vi "dark int time.vi"(8 "error in (no error)":errorcluster) -> (0 "error out":errorcluster, 1 "Stop and Save":bool, 2 "int time":dbl)   [LabVIEW 2013]
uses:
  <vilib>/Utility/file.llb/Read From Spreadsheet File (DBL).vi
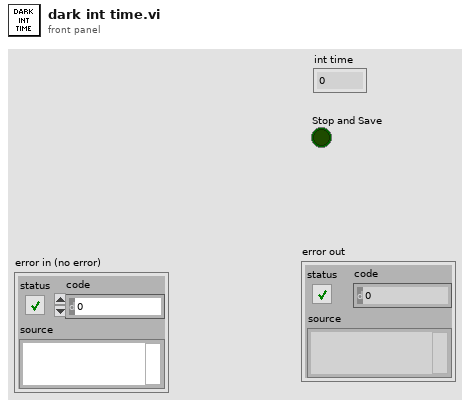
[diagram p1: front panel]
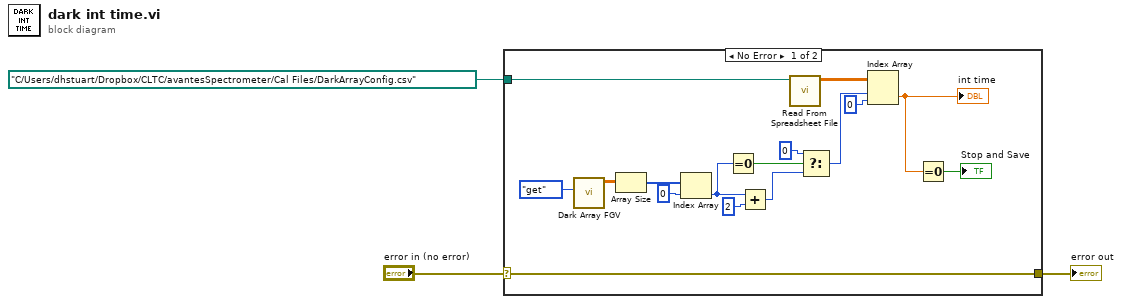
[diagram p0: block diagram]
diagram:
  n1 = case shown="No Error" "error in (no error)" {
    selector: "error in (no error)" -> [w6 w20]
    tunnel: path "C:/Users/dhstuart/Dropbox/CLTC/avantesSpectrometer/Cal Files/DarkArrayConfig.csv" ("file path (dialog if empty)") -> [w19 _]
    tunnel: [w6 w20] -> w1
    frame No Error {
      n2 = call "Dark Array FGV.vi"("Control"=enum16{"get", "add", "reset"}."get") -> ("Out"=w17:dbl[][])  [unwired: 10 in]
      n3 = Array Size(array=w17) -> (size(s)=w16:i32[])
      n4 = Index Array(array=w16, index=0) -> (element=w10:i32)
      n5 = Equal To 0?(x=w10) -> (x = 0?=w11:bool)
      n6 = Add(x=w10, y=2) -> (x+y=w9:i32)
      n7 = call-poly <vilib>:"Read From Spreadsheet File.vi"("file path (dialog if empty)"=w19) -> ("all rows"=w14:dbl[][])  [unwired: 6 in, 4 out]
      n8 = Select(t=0, s=w11, f=w9) -> (s? t:f=w7:i32)
      n9 = Index Array(array=w14, index (row)=w7, index (col)=0 ("disabled index (col)")) -> (element=w5:dbl)
      "int time" <- w5
      n10 = Equal To 0?(x=w5) -> (x = 0?=→"Stop and Save":bool)
    }
    frame Error {
    }
  }
  "error out" <- w1
